vi "Coincidence hunt limit.vi"() -> ()   [LabVIEW 2016]
panel:
  in  "Coinchunt Lim":i32
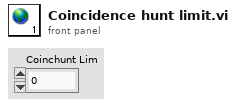
[diagram p1: front panel]
diagram:
